vi "Periodic Tasks.vi"(8 "error in":errorcluster) -> ()   [LabVIEW 2016]
doc: "This VI runs in parallel to other tasks. It can contain as many user-defined periodic loops as you need. These can carry out PID or other sorts of timed response."
uses:
  Robot Global Data.vi
  <vilib>/Rock Robotics/Network Tables/NT Write Number.vi
  <vilib>/Rock Robotics/WPI/Solenoid/WPI_SolenoidValue.ctl
panel:
  out "error out":errorcluster
  out "Left Sensor Position":dbl
  out "Left Sensor Velocity":dbl
  out "Right Sensor Position":dbl
  out "Right Sensor Velocity":dbl
  out "Right Encoder Velocity":dbl
  out "Right Encoder Position":dbl
  out "Left Encoder Velocity":dbl
  out "Left Encoder Position":dbl
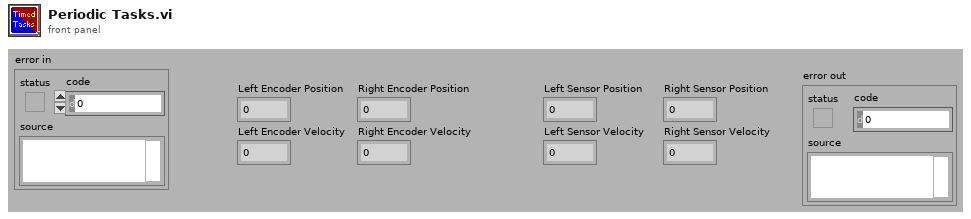
[diagram p1: front panel]
types:
  T1 = typedef "WPI_SolenoidValue.ctl" = enum16{"Off", "On", "Forward", "Reverse"}
  T2 = typedef "WPI_AccelerometerDevRef.ctl" = cluster{"DevStatus":errorcluster, "Scaling":T3, "Analog Channels":T4, "I2C Bus":T6, "SPI Bus":T7, "Accel Range":T8, "ADXL Axes":T9, "Handle":i32, "Device Address":u8, "Accel Type":enum16{"Analog", "ADXL345 I2C", "ADXL345 SPI", "Internal", "ADXL362 SPI"}}
  T3 = typedef "WPI_AccelerometerScaling.ctl" = cluster{"Gain (VoltsPerG)":dbl, "Center Voltage":dbl}
  T4 = typedef "WPI_AccelerometerAnalogChannels.ctl" = cluster{"X-Axis":T5, "Y-Axis":T5, "Z-Axis":T5}
  T5 = typedef "FPGA_AIChannel.ctl" = enum8{"AI 0", "AI 1", "AI 2", "AI 3", "AI MXP 0", "AI MXP 1", "AI MXP 2", "AI MXP 3", "Invalid"}
  T6 = typedef "i2c_bus.ctl" = enum16{"I2C On-Board", "I2C MXP", "Invalid"}
  T7 = typedef "spi_bus.ctl" = enum16{"SPI On-Board, CS0", "SPI On-Board, CS1", "SPI On-Board, CS2", "SPI On-Board, CS3", "SPI MXP", "Invalid"}
  T8 = typedef "ADXL345 Range.ctl" = u8
  T9 = typedef "WPI_AccelerometerADXL345 Axes.ctl" = cluster{"X-Axis":bool, "Y-Axis":bool, "Z-Axis":bool}
  T10 = cluster{"X-Axis":dbl, "Y-Axis":dbl, "Z-Axis":dbl}
  T11 = typedef "WPI_JoystickDevRef.ctl" = cluster{"Device":T12}
  T12 = typedef "WPI_JoystickDeviceEnum.ctl" = enum16{"USB 0", "USB 1", "USB 2", "USB 3", "USB 4", "USB 5"}
  T13 = typedef "WPI_MotorControlDeviceRef.ctl" = cluster{"DeviceStatus":errorcluster, "Type":T14, "PWM":cluster{"PWM Channel":T15, "DeadBand":T16}, "CAN":cluster{"Device Number":u8, "SetOutput VI Ref":variant, "GetOutput VI Ref":variant, "Enable VI Ref":variant, "Disable VI Ref":variant, "Data":variant}, "Invert":bool}
  T14 = typedef "WPI_MotorControlType.ctl" = enum16{"PWM", "CAN"}
  T15 = typedef "FPGA_DIOPWMChannel.ctl" = enum8{"PWM 0", "PWM 1", "PWM 2", "PWM 3", "PWM 4", "PWM 5", "PWM 6", "PWM 7", "PWM 8", "PWM 9", "PWM MXP 0", "PWM MXP 1", "PWM MXP 2", "PWM MXP 3", "PWM MXP 4", "PWM MXP 5", "PWM MXP 6", "PWM MXP 7", "PWM MXP 8", "PWM MXP 9", "Invalid"}
  T16 = typedef "WPI_PWMDeadband.ctl" = cluster{"Name":string, "maxPositivePwm":i32, "minPositivePwm":i32, "centerPwm":i32, "maxNegativePwm":i32, "minNegativePwm":i32, "angularRange":u16}
  T17 = typedef "WPI_CANTalonSRX_GlobalStatus.ctl" = cluster{"Applied Throttle":dbl, "Module Enabled":bool, "CAN Error":errorcluster, "Closed Loop Error":dbl, "Forward Limit Switch Closed":bool, "Reverse Limit Switch Closed":bool, "Sensor Position":dbl, "Sensor Velocity":dbl, "Current":dbl, "Sticky Fault - Over Temp":bool, "Sticky Fault - Under Voltage":bool, "Sticky Fault - Forward Limit":bool, "Sticky Fault - Reverse Limit":bool, "Sticky Fault - Forward Soft Limit":bool, "Sticky Fault - Reverse Soft Limit":bool, "Brake is Enabled":bool, "Encoder Position":dbl, "Encoder Velocity":dbl, "Encoder Index Count":dbl, "Encoder A Pin State":bool, "Encoder B Pin State":bool, "Encoder Index Pin State":bool, "Analog In":dbl, "Analog In Velocity":dbl, "Temperature (C)":dbl, "Battery Voltage":dbl, "Control 5 Is Supported":bool, "Current Profile Slot Select":dbl, "Pos Div 8":bool, "Vel Div 4":bool, "Pulse Width Position":i32, "Pulse Width Velocity":i32, "Pulse Width Rise To Rise (us)":i32, "Pulse Width Rise To Fall (us)":i32, "Mot Prof Active Is Under Run":bool, "Mot Prof Active Has Under Run":bool, "Mot Prof Active Is Last":bool, "Mot Prof Active Velocity Only":bool, "Mot Prof Active Is Valid":bool, "Mot Prof Buffer Is Full":bool, "Mot Prof Active Profile Slot Select":i32, "Mot Prof NextID":i32, "Mot Prof Count":i32, "Mot Prof Active Velocity":dbl, "Mot Prof Active Position":dbl, "Mot Prof Output Enable":i32}
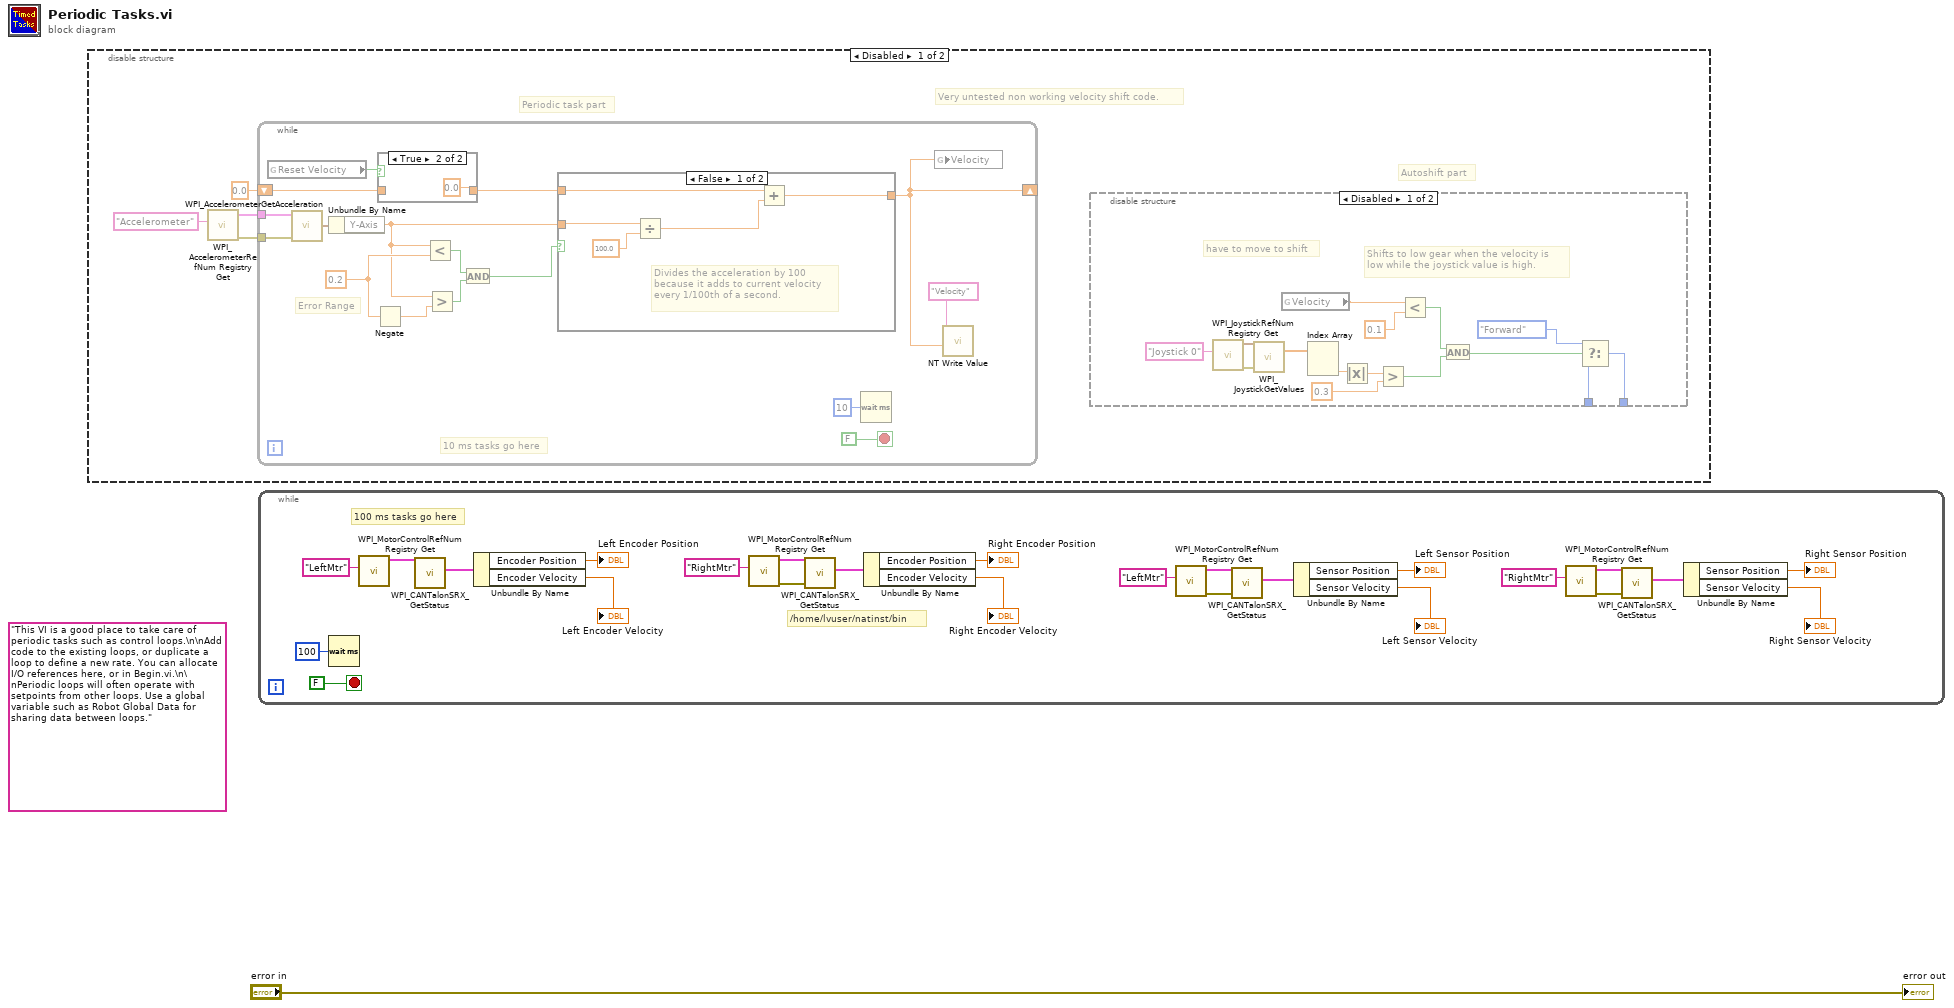
[diagram p0: block diagram]
diagram:
  (unwired) "This VI is a good place to take care of periodic tasks such as control loops.\n\nAdd code to the existing loops, or duplicate a loop to define a new rate. You can allocate I/O references here, or in Begin.vi.\n\nPeriodic loops will often operate with setpoints from other loops. Use a global variable such as Robot Global Data for sharing data between loops."
  # "/home/lvuser/natinst/bin"
  n1 = disable-structure shown="Disabled" {
    frame Disabled {
      # "Periodic task part"
      # "Autoshift part"
      # "Very untested non working velocity shift code."
      n2 = call <vilib>:"WPI_AccelerometerRefNum Registry Get.vi"("refnum name"="Accelerometer") -> ("error out"=w4:errorcluster, "AccelerometerDevRef"=w5:T2)  [unwired: 9 in]
      n3 = while {
        tunnel: w5 -> [w34]
        tunnel: w4 -> [w33]
        shift-right: [w21] -> _
        shift-left: 0.0 -> [w24]
        stop <- FALSE stop-if-true
        w30 = 0.2 ("y")
        # "10 ms tasks go here"
        # "Error Range"
        n4 = global read "Robot Global Data.vi" "Reset Velocity"() -> (w23:bool)
        n5 = call <vilib>:"WPI_AccelerometerGetAcceleration.vi"("error in"=w33, "AccelerometerDevRef"=w34) -> ("Accelerations"=w32:T10)  [unwired: 7 in, 2 out]
        n6 = Unbundle By Name(w32) -> ("Y-Axis"=w26:dbl)
        n7 = Negate(x=w30) -> (-x=w31:dbl)
        n8 = case shown="True" w23 {
          tunnel: [w37 0.0] -> w25
          tunnel: w24 -> [w37 _]
          frame False {
          }
          frame True {
          }
        }
        n9 = Less?(x=w26, y=w30) -> (x < y?=w29:bool)
        n10 = Greater?(x=w26, y=w31) -> (0:w28:bool)
        n11 = And(x=w29, y=w28) -> (x .and. y?=w27:bool)
        n12 = case shown="False" w27 {
          tunnel: w26 -> [w41 _]
          tunnel: [w42 w44] -> w21
          tunnel: w25 -> [w43 w44]
          frame False {
            # "Divides the acceleration by 100\nbecause it adds to current velocity \nevery 1/100th of a second."
            n13 = Divide(x=w41, y=100.0) -> (x/y=w40:dbl)
            n14 = Add(x=w43, y=w40) -> (x+y=w42:dbl)
          }
          frame True {
          }
        }
        n15 = Wait (ms)(milliseconds to wait=u32 10) -> ()  [unwired: 1 out]
        n16 = global write "Robot Global Data.vi" "Velocity"(w21) -> ()
        n17 = call-poly <vilib>:"NT Write Value.vi"("Numeric"=w21, "Name"="Velocity") -> ()  [unwired: 9 in, 1 out]
      }
      n18 = disable-structure shown="Disabled" {
        disable-tunnel: _ -> [w20 _]
        disable-tunnel: [w19 _] -> _
        frame Disabled {
          # "have to move to shift"
          # "Shifts to low gear when the velocity is \nlow while the joystick value is high."
          n19 = call <vilib>:"WPI_JoystickRefNum Registry Get.vi"("refnum name"="Joystick 0") -> ("error out"=w17:errorcluster, "JoystickDevRef"=w16:T11)  [unwired: 9 in]
          n20 = call <vilib>:"WPI_JoystickGetValues.vi"("error in (no error)"=w17, "JoystickDevRef"=w16) -> ("Axes"=w15:dbl[])  [unwired: 5 in, 4 out]
          n21 = global read "Robot Global Data.vi" "Velocity"() -> (w6:dbl)
          n22 = Index Array(array=w15) -> (element #2=w14:dbl)  [unwired: 2 in, 1 out]
          n23 = Absolute Value(x=w14) -> (abs(x)=w13:dbl)
          n24 = Greater?(x=w13, y=0.3) -> (0:w9:bool)
          n25 = Less?(x=w6, y=0.1) -> (x < y?=w10:bool)
          n26 = And(x=w10, y=w9) -> (x .and. y?=w8:bool)
          n27 = Select(t=WPI_SolenoidValue."Forward", s=w8, f=w20) -> (s? t:f=w19:T1)
        }
        frame Enabled {
        }
      }
    }
    frame Enabled {
    }
  }
  n28 = while {
    stop <- FALSE stop-if-true
    # "100 ms tasks go here"
    n29 = Wait (ms)(milliseconds to wait=u32 100) -> ()  [unwired: 1 out]
    n30 = call <vilib>:"WPI_MotorControlRefNum Registry Get.vi"("refnum name"="LeftMtr") -> ("MotorControlDevRef"=w63:T13)  [unwired: 9 in, 1 out]
    n31 = call <vilib>:"WPI_CANTalonSRX_GetStatus.vi"("CAN Talon SRX Ref"=w63) -> ("Talon SRX Status"=w61:T17)  [unwired: 8 in, 2 out]
    n32 = Unbundle By Name(w61) -> ("Encoder Position"=→"Left Encoder Position":dbl, "Encoder Velocity"=→"Left Encoder Velocity":dbl)
    n33 = call <vilib>:"WPI_MotorControlRefNum Registry Get.vi"("refnum name"="RightMtr") -> ("error out"=w55:errorcluster, "MotorControlDevRef"=w56:T13)  [unwired: 9 in]
    n34 = call <vilib>:"WPI_CANTalonSRX_GetStatus.vi"("error in (no error)"=w55, "CAN Talon SRX Ref"=w56) -> ("Talon SRX Status"=w58:T17)  [unwired: 7 in, 2 out]
    n35 = Unbundle By Name(w58) -> ("Encoder Position"=→"Right Encoder Position":dbl, "Encoder Velocity"=→"Right Encoder Velocity":dbl)
    n36 = call <vilib>:"WPI_MotorControlRefNum Registry Get.vi"("refnum name"="LeftMtr") -> ("error out"=w45:errorcluster, "MotorControlDevRef"=w46:T13)  [unwired: 9 in]
    n37 = call <vilib>:"WPI_CANTalonSRX_GetStatus.vi"("error in (no error)"=w45, "CAN Talon SRX Ref"=w46) -> ("Talon SRX Status"=w48:T17)  [unwired: 7 in, 2 out]
    n38 = Unbundle By Name(w48) -> ("Sensor Position"=→"Left Sensor Position":dbl, "Sensor Velocity"=→"Left Sensor Velocity":dbl)
    n39 = call <vilib>:"WPI_MotorControlRefNum Registry Get.vi"("refnum name"="RightMtr") -> ("error out"=w54:errorcluster, "MotorControlDevRef"=w53:T13)  [unwired: 9 in]
    n40 = call <vilib>:"WPI_CANTalonSRX_GetStatus.vi"("error in (no error)"=w54, "CAN Talon SRX Ref"=w53) -> ("Talon SRX Status"=w51:T17)  [unwired: 7 in, 2 out]
    n41 = Unbundle By Name(w51) -> ("Sensor Position"=→"Right Sensor Position":dbl, "Sensor Velocity"=→"Right Sensor Velocity":dbl)
  }
  "error out" <- "error in"
